vi "2_1_MNIST_Eval(CPU,GPU).vi"() -> ()   [LabVIEW 2020]
uses:
  Controls/Img_GrayScale.ctl
  <vilib>/Ngene/Deep Learning Toolkit/Toolkit/NN_Network/Controls/NN_Device.ctl
  <vilib>/Ngene/Deep Learning Toolkit/Toolkit/NN_Network/Controls/NN_Save_Before_Destroy_Options.ctl
  <vilib>/Ngene/Deep Learning Toolkit/Toolkit/NN_Network/subVIs/NN_Predict/NN_Predict(In3D_Out1D).vi
  <vilib>/Ngene/Deep Learning Toolkit/Toolkit/NN_Train/Eval_Loss/NN_Eval_Test_Error_Loss/NN_Eval(In3D_Out1D).vi
  <vilib>/Ngene/Deep Learning Toolkit/Toolkit/NN_Train/Eval_Loss/NN_Calc_Cofusion_Matrix/NN_Calc_Confusion_Matrix(In3D_Out1D).vi
  <vilib>/Ngene/Deep Learning Toolkit/Toolkit/Deep_Learning_Toolkit_by_Ngene.lvlib
panel:
  in  "NN_Device":T1
  out "Incorrectly Classified Samples":T2[][](array[typedef])=[[{"image"=array28x28[784 elements], "Truth"=4, "Predicted"=9}, {"image"=array28x28[784 elements], "Truth"=2, "Predicted"=7}, {"image"=array28x28[784 elements], "Truth"=5, "Predicted"=3}, {"image"=array28x28[784 elements], "Truth"=9, "Predicted"=8}, {"image"=array28x28[784 elements], "Truth"=8, "Predicted"=9}, {"image"=array28x28[784 elements], "Truth"=8, "Predicted"=2}, {"image"=array28x28[784 elements], "Truth"=2, "Predicted"=1}, {"image"=array28x28[784 elements], "Truth"=5, "Predicted"=3}, {"image"=array28x28[784 elements], "Truth"=8, "Predicted"=9}, {"image"=array28x28[784 elements], "Truth"=1, "Predicted"=3}], [{"image"=array28x28[784 elements], "Truth"=6, "Predicted"=5}, {"image"=array28x28[784 elements], "Truth"=9, "Predicted"=4}, {"image"=array28x28[784 elements], "Truth"=4, "Predicted"=9}, {"image"=array28x28[784 elements], "Truth"=9, "Predicted"=5}, {"image"=array28x28[784 elements], "Truth"=7, "Predicted"=1}, {"image"=array28x28[784 elements], "Truth"=5, "Predicted"=3}, {"image"=array28x28[784 elements], "Truth"=9, "Predicted"=0}, {"image"=array28x28[784 elements], "Truth"=9, "Predicted"=3}, {"image"=array28x28[784 elements], "Truth"=5, "Predicted"=3}, {"image"=array28x28[784 elements], "Truth"=8, "Predicted"=3}], [{"image"=array28x28[784 elements], "Truth"=9, "Predicted"=4}, {"image"=array28x28[784 elements], "Truth"=5, "Predicted"=3}, {"image"=array28x28[784 elements], "Truth"=7, "Predicted"=9}, {"image"=array28x28[784 elements], "Truth"=6, "Predicted"=0}, {"image"=array28x28[784 elements], "Truth"=9, "Predicted"=8}, {"image"=array28x28[784 elements], "Truth"=4, "Predicted"=9}, {"image"=array28x28[784 elements], "Truth"=9, "Predicted"=8}, {"image"=array28x28[784 elements], "Truth"=9, "Predicted"=4}, {"image"=array28x28[784 elements], "Truth"=2, "Predicted"=4}, {"image"=array28x28[784 elements], "Truth"=5, "Predicted"=3}], [{"image"=array28x28[784 elements], "Truth"=6, "Predicted"=1}, {"image"=array28x28[784 elements], "Truth"=8, "Predicted"=0}, {"image"=array28x28[784 elements], "Truth"=3, "Predicted"=2}, {"image"=array28x28[784 elements], "Truth"=5, "Predicted"=3}, {"image"=array28x28[784 elements], "Truth"=6, "Predicted"=0}, {"image"=array28x28[784 elements], "Truth"=9, "Predicted"=7}, {"image"=array28x28[784 elements], "Truth"=1, "Predicted"=2}, {"image"=array28x28[784 elements], "Truth"=7, "Predicted"=9}, {"image"=array28x28[784 elements], "Truth"=7, "Predicted"=2}, {"image"=array28x28[784 elements], "Truth"=6, "Predicted"=0}], [{"image"=array28x28[784 elements], "Truth"=6, "Predicted"=4}, {"image"=array28x28[784 elements], "Truth"=5, "Predicted"=0}, {"image"=array28x28[784 elements], "Truth"=7, "Predicted"=1}, {"image"=array28x28[784 elements], "Truth"=5, "Predicted"=3}, {"image"=array28x28[784 elements], "Truth"=9, "Predicted"=4}, {"image"=array28x28[784 elements], "Truth"=2, "Predicted"=7}, {"image"=array28x28[784 elements], "Truth"=6, "Predicted"=8}, {"image"=array28x28[784 elements], "Truth"=3, "Predicted"=5}, {"image"=array28x28[784 elements], "Truth"=8, "Predicted"=3}, {"image"=array28x28[784 elements], "Truth"=5, "Predicted"=3}], [{"image"=array28x28[784 elements], "Truth"=3, "Predicted"=8}, {"image"=array28x28[784 elements], "Truth"=9, "Predicted"=3}, {"image"=array28x28[784 elements], "Truth"=9, "Predicted"=8}, {"image"=array28x28[784 elements], "Truth"=9, "Predicted"=8}, {"image"=array28x28[784 elements], "Truth"=9, "Predicted"=7}, {"image"=array28x28[784 elements], "Truth"=7, "Predicted"=1}, {"image"=array28x28[784 elements], "Truth"=0, "Predicted"=7}, {"image"=array28x28[784 elements], "Truth"=8, "Predicted"=2}, {"image"=array28x28[784 elements], "Truth"=2, "Predicted"=7}, {"image"=array28x28[784 elements], "Truth"=6, "Predicted"=2}], [{"image"=array28x28[784 elements], "Truth"=8, "Predicted"=6}, {"image"=array28x28[784 elements], "Truth"=7, "Predicted"=2}, {"image"=array28x28[784 elements], "Truth"=7, "Predicted"=2}, {"image"=array28x28[784 elements], "Truth"=0, "Predicted"=8}, {"image"=array28x28[784 elements], "Truth"=2, "Predicted"=7}, {"image"=array28x28[784 elements], "Truth"=5, "Predicted"=6}, {"image"=array28x28[784 elements], "Truth"=4, "Predicted"=9}, {"image"=array28x28[784 elements], "Truth"=5, "Predicted"=6}, {"image"=[], "Truth"=0, "Predicted"=0}, {"image"=[], "Truth"=0, "Predicted"=0}]]
  in  "Dataset":path
  out "Confusion Matrix":string[][](table)=[["978", "0", "0", "0", "0", "0", "0", "1", "1", "0", "0.9980"], ["0", "1133", "1", "1", "0", "0", "0", "0", "0", "0", "0.9982"], ["0", "1", "1026", "0", "1", "0", "0", "4", "0", "0", "0.9942"], ["0", "0", "1", "1007", "0", "1", "0", "0", "1", "0", "0.9970"], ["0", "0", "0", "0", "978", "0", "0", "0", "0", "4", "0.9959"], ["1", "0", "0", "9", "0", "880", "2", "0", "0", "0", "0.9865"], ["3", "1", "1", "0", "1", "1", "950", "0", "1", "0", "0.9916"], ["0", "3", "3", "0", "0", "0", "0", "1020", "0", "2", "0.9922"], ["1", "0", "2", "2", "0", "0", "1", "0", "966", "2", "0.9918"], ["1", "0", "0", "2", "4", "1", "0", "2", "5", "994", "0.9851"], ["0.9939", "0.9956", "0.9923", "0.9863", "0.9939", "0.9966", "0.9969", "0.9932", "0.9918", "0.9920", ""]]
  out "Error":sgl=0.0068
  out "Loss":sgl=0.02057273
  in  "Weight File Path":path=path "D:/Ngene/GitHub/deepltk_fpga_examples/1_MNIST_Classification(PXI,sbRIO)/Models/0_Original/MNIST_CNN/MNIST_CNN_weights_24_11_25__15_33_35.bin"
  in  "Configuration File Path":path=path "D:/Ngene/GitHub/deepltk_fpga_examples/1_MNIST_Classification(PXI,sbRIO)/Models/0_Original/MNIST_CNN/MNIST_CNN_net_cfg_24_11_25__15_33_35.cfg"
  # "Overview: This VI is designed to evaluate (measure the accuracy of) the model when executed on CPU.\nRequirements: \n•DeepLTK - Deep Learning Toolkit for LabVIEW (https://www.ngene.co/deep-learning-toolkit-for-labview)\nInstructions:\n1.\tProvide the path to the dataset to be evaluated at Dataset. \n2.\tProvide the \"Network Configuration File Path\" and \"Weight File Path\" generated by 0_MNIST(Train).vi\n3.Use NN_Device to specify the device (CPU or GPU) for execution. GPU is applicable only for 64-bit LabVIEW.\n4.\tRun the VI.\n5.\tObserve measured accuracy at Loss, Error and Confusion Matrix indicators, and analyze Incorrectly Classified Samples."
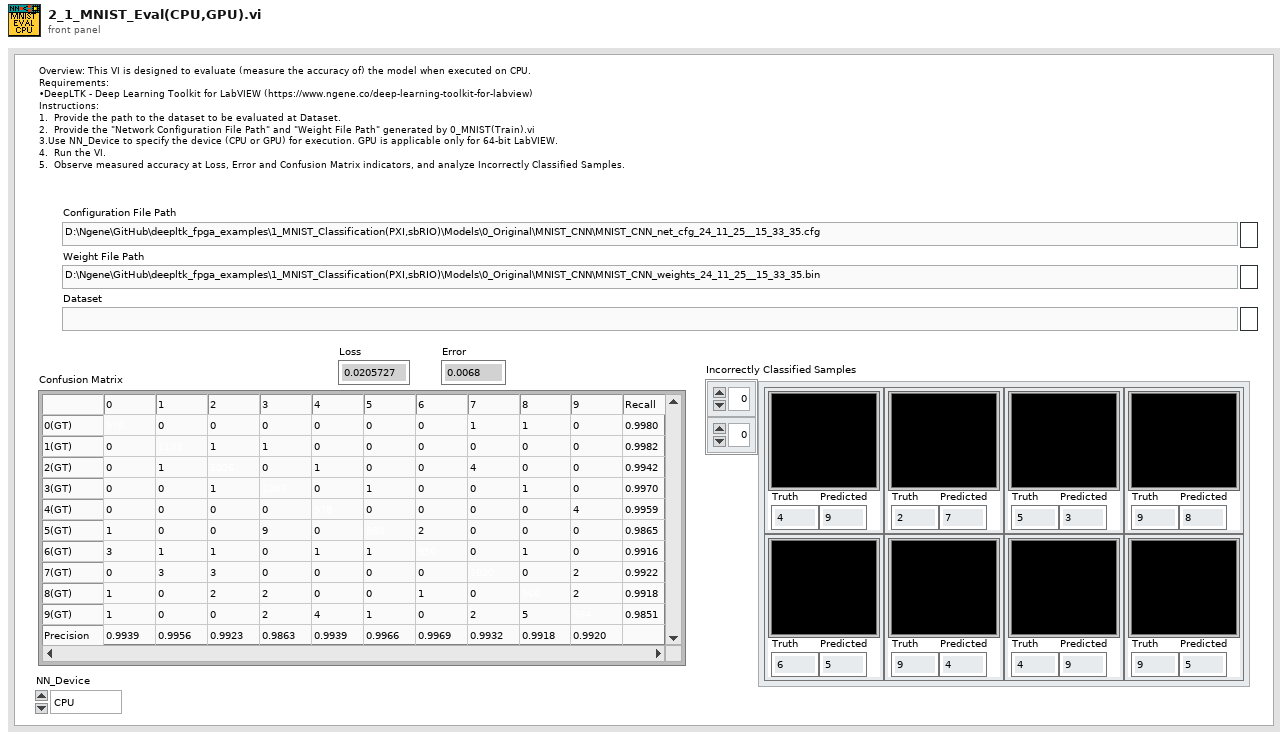
[diagram p1: front panel]
types:
  T1 = typedef "Deep_Learning_Toolkit_by_Ngene.lvlib/NN_Device.ctl" = enum16{"CPU", "GPU"}
  T2 = typedef "Img_GrayScale.ctl" = cluster{"image":sgl[][], "Truth":i32, "Predicted":i32}
  T3 = typedef "Deep_Learning_Toolkit_by_Ngene.lvlib/NN_Save_Before_Destroy_Options.ctl" = cluster{"CFG?":bool, "Weights?":bool, "Render?":bool}
  T4 = typedef "Deep_Learning_Toolkit_by_Ngene.lvlib/NN_DataSets_All(In3D_Out1D).ctl" = cluster{"Train":T5, "Validation":T5, "Test":T5}
  T5 = typedef "Deep_Learning_Toolkit_by_Ngene.lvlib/NN_DataSet(In3D_Out1D).ctl" = cluster{"Inputs Ref.":variant, "Outputs Ref.":T6, "Dataset_Size":i32, "Dims_In":T7, "Dims_Out":i32, "Labels":string[], "File Paths":path[]}
  T6 = typedef "Deep_Learning_Toolkit_by_Ngene.lvlib/NN_Data_ref(2D_SGL).ctl" = refnum<data-value>
  T7 = typedef "Deep_Learning_Toolkit_by_Ngene.lvlib/NN_Dims(C,H,W).ctl" = cluster{"C":i32, "H":i32, "W":i32}
  T8 = typedef "Deep_Learning_Toolkit_by_Ngene.lvlib/NN_Config_Params.ctl" = cluster{"Name":string, "mBatch":i32, "NN_Train_Params":T9, "LR_Decay_Policy":T12, "Labels":string[], "Loss":T14}
  T9 = typedef "Deep_Learning_Toolkit_by_Ngene.lvlib/NN_Train_Params.ctl" = cluster{"Optimizer":T10, "Beta_1":sgl, "Beta_2":sgl, "Weight Decay(L1)":sgl, "Weight Decay(L2)":sgl, "Data_Sampling":T11}
  T10 = typedef "Deep_Learning_Toolkit_by_Ngene.lvlib/NN_Train_Optimizer.ctl" = enum16{"SGD", "Adam", "Adagrad", "Adadelta", "RMSProp", "Nesterov"}
  T11 = typedef "Deep_Learning_Toolkit_by_Ngene.lvlib/NN_Train_Data_Sampling.ctl" = enum16{"Random", "Sequential"}
  T12 = typedef "Deep_Learning_Toolkit_by_Ngene.lvlib/NN_LR_Policy_Cfg.ctl" = cluster{"Policy_Type":T13, "LR0":dbl, "k":sgl, "WarmUp_Policy":enum16{"Step", "Ramp"}, "WarmUp_Iter":i32, "WarmUp_Ratio":sgl}
  T13 = typedef "Deep_Learning_Toolkit_by_Ngene.lvlib/NN_LR_Policy_Type.ctl" = enum16{"Manual", "Step", "Exp", "1/t"}
  T14 = typedef "Deep_Learning_Toolkit_by_Ngene.lvlib/NN_Loss_Config_Params.ctl" = cluster{"Loss_Type":T15, "Loss_Conf_Params":variant}
  T15 = typedef "Deep_Learning_Toolkit_by_Ngene.lvlib/NN_Loss_Type.ctl" = enum16{"None", "MSE", "CrossEntropy", "YOLO_v2", "YOLO_v4"}
  T16 = typedef "Deep_Learning_Toolkit_by_Ngene.lvlib/NN_Layer_Config_Params.ctl" = cluster{"Layer_Type":T17, "Layer_Conf_Params":variant, "Input Layers":string[]}
  T17 = typedef "Deep_Learning_Toolkit_by_Ngene.lvlib/NN_Layer_Type.ctl" = enum16{"Input1D", "Input3D", "Conv1D", "Conv2D", "Conv2D_Adv", "MaxPool", "AvgPool", "UpSample", "DropOut3D", "ShortCut", "Concat", "SoftMax3D", "FC", "DropOut", "Softmax", "Flatten", "YOLO_v2", "YOLO_v4", "Activation", "BatchNormalization", "Unsupported"}
  T18 = typedef "Deep_Learning_Toolkit_by_Ngene.lvlib/NN.ctl" = cluster{"Name":string, "No of Layers":i32, "mBatch":i32, "Layers":T19[], "Dimty":T20, "Dims_In":T7, "Dims_Out":T7, "Working_Dir":path, "Train?":bool, "Train_Params":T9, "LR_Update_Policy":T12, "Session Data":T21, "Ground_truth":T22, "NNg_hdls":T23, "NN_Device":T1, "GPU Id":i32, "Labels":string[], "Receptive Field":T24[], "Loss_Type":T15, "Loss_Cfg_Prms":variant, "NNG_WS":T25}
  T19 = typedef "Deep_Learning_Toolkit_by_Ngene.lvlib/NN_Layer_ref.ctl" = refnum<data-value>
  T20 = typedef "Deep_Learning_Toolkit_by_Ngene.lvlib/NN_In_Out_Dim-ty.ctl" = enum8{"In1D_Out1D", "In3D_Out1D", "In3D_Out3D", "In3D_OutBBox"}
  T21 = typedef "Deep_Learning_Toolkit_by_Ngene.lvlib/NN_Train_Session_Data.ctl" = cluster{"Epochs":sgl, "Tot_Iter":i32, "LR":sgl, "LR_iter":i32}
  T22 = typedef "Deep_Learning_Toolkit_by_Ngene.lvlib/NN_Ground_truth.ctl" = cluster{"Y":variant}
  T23 = typedef "Deep_Learning_Toolkit_by_Ngene.lvlib/nng_cuda_handles.ctl" = cluster{"cudnn":u64, "cublas":u64, "stream":u64, "curand":u64}
  T24 = typedef "Deep_Learning_Toolkit_by_Ngene.lvlib/NN_Dims(V,H).ctl" = cluster{"V":i32, "H":i32}
  T25 = typedef "Deep_Learning_Toolkit_by_Ngene.lvlib/NNG_WS.ctl" = cluster{"NNG_WS_Mem":T26, "Max_WS_Size":i64}
  T26 = typedef "Deep_Learning_Toolkit_by_Ngene.lvlib/NNg_WS_Mem_DVR.ctl" = refnum<data-value>
  T27 = typedef "Deep_Learning_Toolkit_by_Ngene.lvlib/NN_Eval_Params.ctl" = cluster{"Loss":sgl, "Error":sgl}
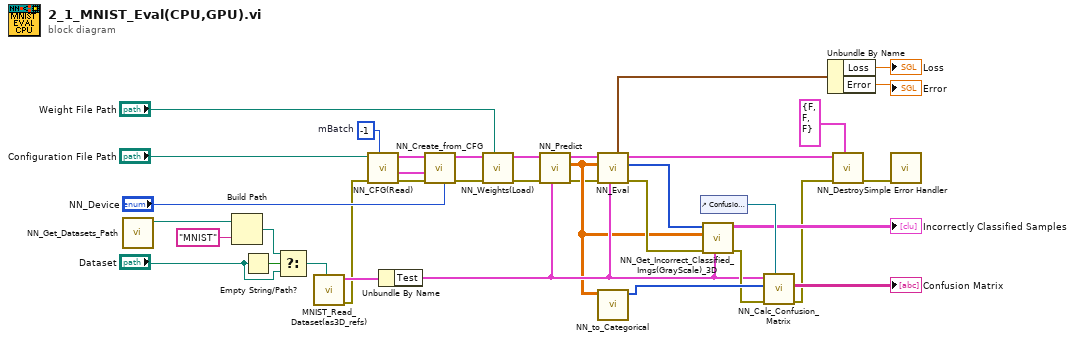
[diagram p0: block diagram]
diagram:
  w21 = -1  # mBatch
  n1 = call "NN_Get_Datasets_Path.vi"() -> ("Datasets path"=w3:path)  [unwired: 11 in]
  n2 = Build Path(base path=w3, name or relative path="MNIST") -> (appended path=w5:path)
  n3 = Empty String/Path?(string/path="Dataset") -> (empty?=w4:bool)
  n4 = Select(t=w5, s=w4, f="Dataset") -> (s? t:f=w2:path)
  n5 = call "MNIST_Read_Dataset(as3D_refs).vi"("MNIST Dataset Path"=w2) -> ("error out"=w8:errorcluster, "Data(3D)_Refs"=w33:T4)  [unwired: 9 in]
  n6 = call <vilib>:"NN_CFG(Read).vi"("mBatch"=w21, "error in (no error)"=w8, "CFG file path"="Configuration File Path") -> ("error out"=w24:errorcluster, "Net_Cfg"=w25:T8, "Layer_Cfg"=w23:T16[])  [unwired: 6 in]
  n7 = Unbundle By Name(w33) -> ("Test"=w15:T5)
  n8 = call <vilib>:"NN_Create_from_CFG.vi"("NN_Device"="NN_Device", "error in (no error)"=w24, "Net_Cfg"=w25, "Layer_Cfg"=w23) -> ("error out"=w26:errorcluster, "NN out"=w22:T18)  [unwired: 6 in]
  n9 = call <vilib>:"NN_Weights(Load).vi"("Weight File Path"="Weight File Path", "error in (no error)"=w26, "NN in"=w22) -> ("error out"=w16:errorcluster, "NN out"=w17:T18)  [unwired: 7 in]
  n10 = call-poly <vilib>:"NN_Predict.vi"("Dataset"=w15, "error in (no error)"=w16, "NN in"=w17) -> ("error out"=w7:errorcluster, "Predictions"=w14:sgl[][], "NN out"=w10:T18)  [unwired: 6 in]
  n11 = call-poly <vilib>:"NN_Eval.vi"("Dataset"=w15, "error in (no error)"=w7, "Predictions"=w14, "NN in"=w10) -> ("error out"=w29:errorcluster, "Incrct_Class_idx"=w30:i32[], "NN out"=w11:T18, "NN_Eval_Params"=w37:T27)  [unwired: 4 in]
  n12 = call <vilib>:"NN_to_Categorical.vi"("Prediction"=w14) -> ("Label_Idx"=w34:i32[])  [unwired: 10 in]
  n13 = control-ref of="Confusion Matrix"() -> (w31:refnum<vi>)
  n14 = call "NN_Get_Incorrect_Classified_Imgs(GrayScale)_3D.vi"("Test_Data"=w15, "error in (no error)"=w29, "Predictions"=w14, "MisClassed_idx"=w30) -> ("error out"=w28:errorcluster, "Images(GrayScale)"=→"Incorrectly Classified Samples":T2[][])  [unwired: 6 in]
  n15 = call-poly <vilib>:"NN_Calc_Confusion_Matrix.vi"("Confusion Matrix (Table) ref."=w31, "error in (no error)"=w28, "Predictions"=w34, "Dataset"=w15) -> ("error out"=w12:errorcluster, "Confusion Matrix (Table)"=→"Confusion Matrix":string[][])  [unwired: 3 in, 3 out]
  n16 = Unbundle By Name(w37) -> ("Loss"=→"Loss":sgl, "Error"=→"Error":sgl)
  n17 = call <vilib>:"NN_Destroy.vi"("Save (T, T, T)"=T3 {"CFG?"=FALSE, "Weights?"=FALSE, "Render?"=FALSE}, "error in (no error)"=w12, "NN in"=w11) -> ("error out"=w9:errorcluster)  [unwired: 7 in, 1 out]
  n18 = call <vilib>:"Simple Error Handler.vi"("error in (no error)"=w9) -> ()  [unwired: 4 in, 5 out]
